vi "Cleanup.vi"(8 "error in (no error)":errorcluster, 11 "Challenge DB in":refnum<class "Challenge DB.lvclass">) -> (0 "error out":errorcluster)   [LabVIEW 2020, in "Summer of LabVIEW.lvlib" / "Challenge DB.lvclass"]
uses:
  Challenge DB.lvclass
  Challenge DB.lvclass/Challenge DB.ctl
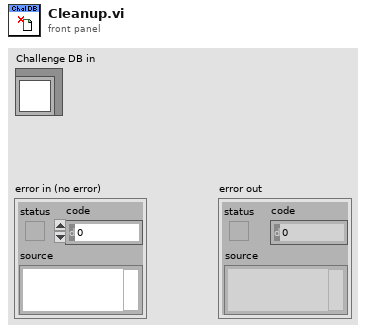
[diagram p1: front panel]
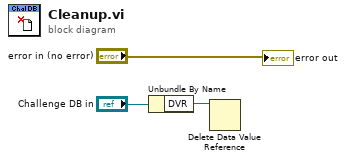
[diagram p0: block diagram]
diagram:
  n1 = Unbundle By Name("Challenge DB in") -> ("DVR"=w1:refnum<data-value>)
  n2 = Delete Data Value Reference(data value reference=w1) -> ()  [unwired: 1 in, 2 out]
  "error out" <- "error in (no error)"
